vi "LVClass_Pupil Read Pupil.vi"(8 "error in (no error)":errorcluster, 11 "Pupil in":refnum<class "Pupil.lvclass">) -> (0 "error out":errorcluster, 2 "Pupil":i32, 3 "Pupil out":refnum<class "Pupil.lvclass">)   [LabVIEW 2020, in "Pupil.lvclass"]
uses:
  Pupil.lvclass
  Pupil.lvclass/Pupil.ctl
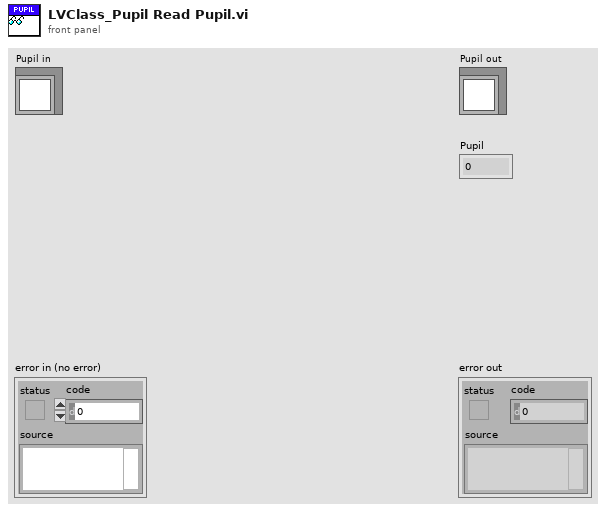
[diagram p1: front panel]
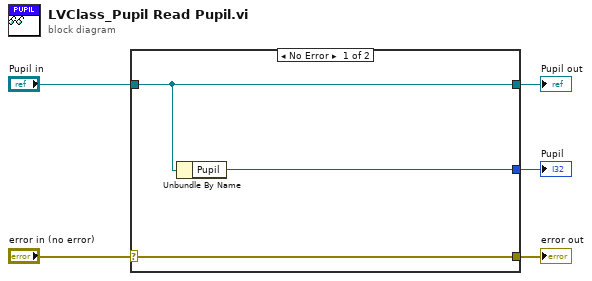
[diagram p0: block diagram]
diagram:
  n1 = case shown="No Error" "error in (no error)" {
    selector: "error in (no error)" -> [w8 w9]
    tunnel: [w8 w9] -> w4
    tunnel: [w7 w10] -> w2
    tunnel: "Pupil in" -> [w7 w10]
    tunnel: [w6 _] -> w1
    frame No Error {
      n2 = Unbundle By Name(w7) -> ("Pupil"=w6:i32)
    }
    frame Error {
    }
  }
  "error out" <- w4
  "Pupil out" <- w2
  "Pupil" <- w1
